vi "create_path.vi"(1 "relative path":string) -> (0 "absolute path":string)   [LabVIEW 2017]
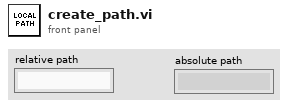
[diagram p1: front panel]
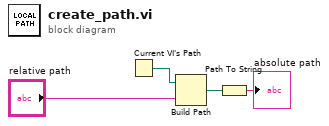
[diagram p0: block diagram]
diagram:
  n1 = Current VI's Path() -> (path=w2:path)
  n2 = Build Path(base path=w2, name or relative path="relative path") -> (appended path=w3:path)
  n3 = Path To String(path=w3) -> (string=→"absolute path":string)
